vi "Measure and Read Value.vi"(6 "Header":string, 7 "Position":u32, 8 "error in (no error)":errorcluster, 9 "Calibration Type":string, 10 "Cree Communications":refnum<class "Cree Communications.lvclass">, 11 "Calibration in":refnum<class "Calibration.lvclass">) -> (0 "error out":errorcluster, 2 "DSpic Measurement":dbl, 3 "Actual Measurement":dbl)   [LabVIEW 2015, in "Calibration.lvclass"]
uses:
  Calibration.lvclass
  Classes/Cree Communications/Class/Cree Communications.lvclass
  Classes/Cree Communications/Cree Comms Messages/Get Vsec Measurement/Get Vsec Measurement.lvclass
  Classes/Cree Communications/Cree Comms Messages/Get ITemp Measurement/Get ITemp Measurement.lvclass
  Classes/Cree Communications/Cree Comms Messages/Get String Current/Get String Current.lvclass
  Classes/Cree Communications/Cree Comms Messages/CC Message/CC Message.lvclass/CC Message.ctl
  Classes/Cree Communications/Cree Comms Messages/CC Message/CC Message.lvclass
  Driver Test/Driver Test.lvclass
  Test Class/Test Class.lvclass
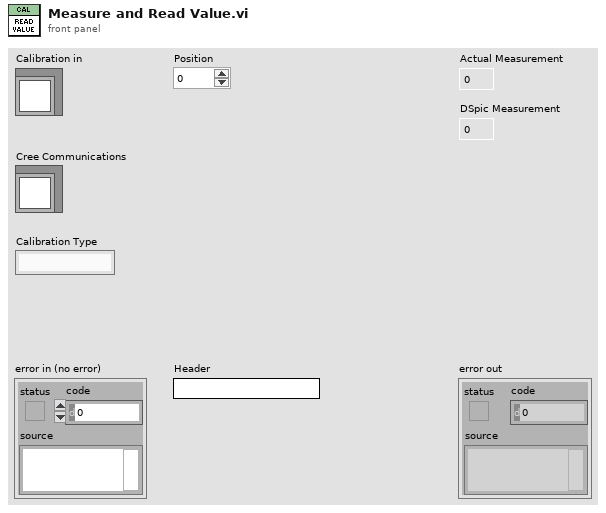
[diagram p1: front panel]
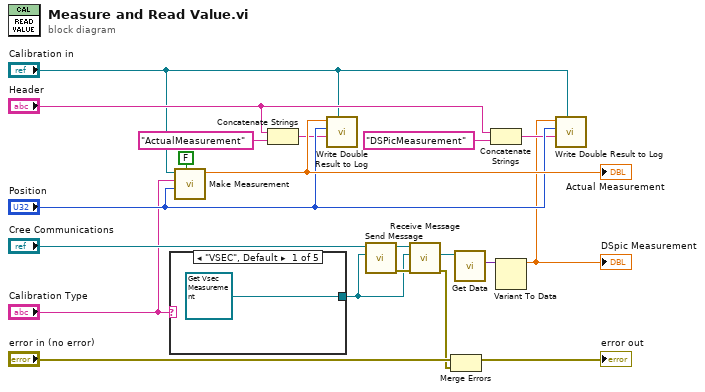
[diagram p0: block diagram]
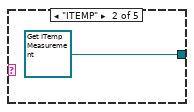
[diagram p2: hidden frame]
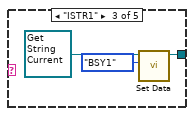
[diagram p3: hidden frame]
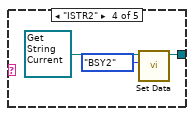
[diagram p4: hidden frame]
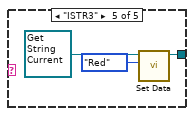
[diagram p5: hidden frame]
diagram:
  n1 = case shown="\"VSEC\", Default" "Calibration Type" {
    tunnel: [refnum<class "Get Vsec Measurement.lvclass"> refnum ("Cree Comms Messages.lvlib:Get Vsec Measurement.lvclass") refnum<class "Get ITemp Measurement.lvclass"> refnum ("Cree Comms Messages.lvlib:Get ITemp Measurement.lvclass") w25 w28 w31] -> w15
    frame "VSEC", Default {
    }
    frame "ITEMP" {
    }
    frame "ISTR1" {
      n2 = call "Set Data.vi"("Data"=enum16{"Red", "BSY1", "BSY2"}."BSY1" ("Message Type"), "CC Message in"=refnum<class "Get String Current.lvclass"> refnum ("Cree Comms Messages.lvlib:Get String Current.lvclass")) -> ("CC Message out"=w25:refnum<class "Get String Current.lvclass">)  [unwired: 8 in, 1 out]
    }
    frame "ISTR2" {
      n3 = call "Set Data.vi"("Data"=enum16{"Red", "BSY1", "BSY2"}."BSY2" ("Message Type"), "CC Message in"=refnum<class "Get String Current.lvclass"> refnum ("Cree Comms Messages.lvlib:Get String Current.lvclass")) -> ("CC Message out"=w28:refnum<class "Get String Current.lvclass">)  [unwired: 8 in, 1 out]
    }
    frame "ISTR3" {
      n4 = call "Set Data.vi"("Data"=enum16{"Red", "BSY1", "BSY2"}."Red" ("Message Type"), "CC Message in"=refnum<class "Get String Current.lvclass"> refnum ("Cree Comms Messages.lvlib:Get String Current.lvclass")) -> ("CC Message out"=w31:refnum<class "Get String Current.lvclass">)  [unwired: 8 in, 1 out]
    }
  }
  n5 = call "Make Measurement.vi"("Record Result (True)"=FALSE, "Position"="Position", "Channel"="Calibration Type", "Driver Test in"="Calibration in") -> ("Value"=w20:dbl)  [unwired: 6 in, 1 out]
  "Actual Measurement" <- w20
  n6 = Concatenate Strings("Header", "ActualMeasurement" ("string")) -> (w2:string)
  n7 = call "Write Double Result to Log.vi"("Test Class in"="Calibration in", "Label"=w2, "Position"="Position", "Value"=w20) -> ()  [unwired: 7 in, 1 out]
  n8 = call "Send Message.vi"("Cree Comms Message"=w15, "Acrobat Template in"="Cree Communications") -> ("error out"=w16:errorcluster, "Acrobat Template out"=w17:refnum<class "Cree Communications.lvclass">)  [unwired: 8 in]
  n9 = call "Receive Message.vi"("error in (no error)"=w16, "CC Message"=w15, "Acrobat Template in"=w17) -> ("error out"=w7:errorcluster, "Cree Comms Message"=w14:refnum<class "CC Message.lvclass">)  [unwired: 6 in, 1 out]
  n10 = Merge Errors("error in (no error)", w7) -> (→"error out":errorcluster)
  n11 = call "Get Data.vi"("CC Message in"=w14) -> ("Data"=w13:variant)  [unwired: 8 in, 2 out]
  n12 = Concatenate Strings("Header", "DSPicMeasurement" ("string")) -> (w6:string)
  n13 = Variant To Data(Variant=w13) -> (data=w5:dbl)  [unwired: 2 in, 1 out]
  "DSpic Measurement" <- w5
  n14 = call "Write Double Result to Log.vi"("Test Class in"="Calibration in", "Label"=w6, "Position"="Position", "Value"=w5) -> ()  [unwired: 7 in, 1 out]
